vi "Kinect - Land (SubVI).vi"(8 "error in (no error)":errorcluster, 11 "Array of Joint Positions Out":dbl[][](array[numeric])) -> (0 "error out":errorcluster, 1 "Absolute Distance Between Joints":dbl(knob)=0.1448702604855027 scale=0.0..1.5, 2 "Boolean":bool, 3 "Array of Joint Positions Out 2":dbl[][](array[numeric]))   [LabVIEW 2014]
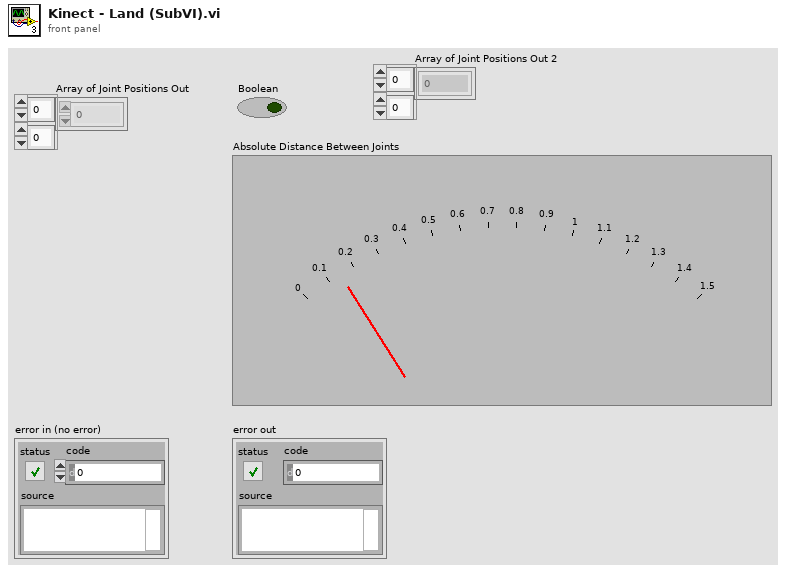
[diagram p1: front panel]
types:
  T1 = enum16{"hip centre", "spine", "shoulder centre", "head", "shoulder left", "elbow left", "wrist left", "hand left", "shoulder right", "elbow right", "wrist right", "hand right", "hip left", "knee left", "ankle left", "foot left", "hip right", "knee right", "ankle right", "foot right"}
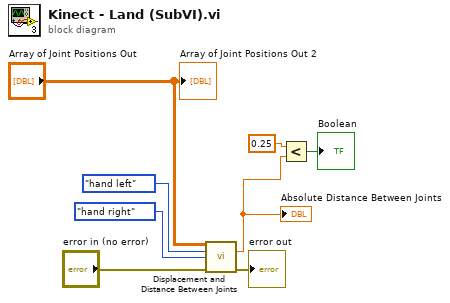
[diagram p0: block diagram]
diagram:
  n1 = call <vilib>:"Displacement and Distance Between Joints.vi"("Array of Joint Positions"="Array of Joint Positions Out", "Joint 1"=T1."hand left", "Joint 2"=T1."hand right", "error in (no error)"="error in (no error)") -> ("Absolute Distance Between Joints"=w1:dbl, "error out"=→"error out":errorcluster)  [unwired: 9 in, 1 out]
  "Absolute Distance Between Joints" <- w1
  n2 = Less?(x=0.25 ("Minimal distance"), y=w1) -> (x < y?=→"Boolean":bool)
  "Array of Joint Positions Out 2" <- "Array of Joint Positions Out"
